vi "Save Notebook Rich Text Box.vi"(6 "Backup?":bool, 8 "Error In":errorcluster, 9 "Dialog (F)":bool, 10 "File Path Control":path, 11 ".NET Refnum in":refnum<k24>) -> (0 "Error Out":errorcluster, 1 "cancelled":bool, 2 "File Path out":path)   [LabVIEW 2019, in "Notebook.lvlib"]
uses:
  Notebook.lvlib
  System.Windows.Forms
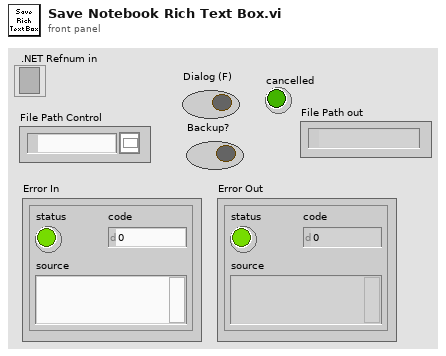
[diagram p1: front panel]
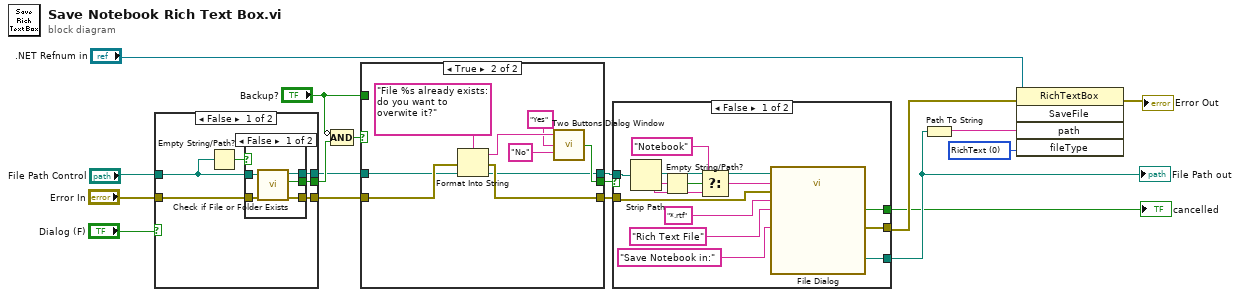
[diagram p0: block diagram]
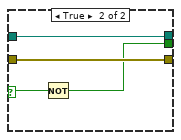
[diagram p5: hidden frame]
diagram:
  w10 = 0 items=["RichText", "PlainText", "RichNoOleObjs", "TextTextOleObjs", "UnicodePlainText"] ("fileType")
  n1 = case shown="False" "Dialog (F)" {
    selector: "Dialog (F)" -> [_ w35]
    tunnel: "File Path Control" -> [w21 w32]
    tunnel: "Error In" -> [w24 w34]
    tunnel: [w23 w34] -> w5
    tunnel: [w22 w33] -> w8
    tunnel: [w19 w32] -> w7
    frame False {
      n2 = Empty String/Path?(string/path=w21) -> (empty?=w20:bool)
      n3 = case shown="False" w20 {
        tunnel: w24 -> [w29 w31]
        tunnel: [w28 w31] -> w23
        tunnel: [w27 _] -> w22
        tunnel: w21 -> [w26 w30]
        tunnel: [w25 w30] -> w19
        frame False {
          n4 = call <vilib>:"Check if File or Folder Exists.vi"("error in (no error)"=w29, "path"=w26) -> ("error out"=w28:errorcluster, "file or folder exists?"=w27:bool, "dup path"=w25:path)  [unwired: 7 in]
        }
        frame True {
        }
      }
    }
    frame True {
      n5 = Not(x=w35) -> (.not. x?=w33:bool)
    }
  }
  n6 = Compound Arithmetic op=AND(invert "Backup?", w8) -> (w2:bool)
  n7 = case shown="True" w2 {
    tunnel: w7 -> [w38 w39]
    tunnel: [w38 w39] -> w6
    tunnel: w5 -> [w37 w44]
    tunnel: [w37 w43] -> w4
    tunnel: [w36 w40] -> w3
    tunnel: "Backup?" -> [w36 _]
    frame False {
    }
    frame True {
      n8 = Format Into String(format string="File %s already exists: do you want to overwite it?", error in=w44, w39) -> (resulting string=w45:string, error out=w43:errorcluster)  [unwired: 1 in]
      n9 = call "Two Buttons Dialog Window.vi"("Cancel Button Text"="No" ("F button name (\"Cancel\")"), "OK Button Text"="Yes" ("T button name (\"OK\")"), "Message"=w45) -> ("OK?"=w40:bool)
    }
  }
  n10 = case shown="False" w3 {
    tunnel: [w58 w60] -> w12
    tunnel: [w57 w61] -> w17
    tunnel: w6 -> [w56 w60]
    tunnel: w4 -> [w55 w61]
    tunnel: [w53 _] -> w11
    frame False {
      n11 = Strip Path(path=w56) -> (stripped path=w54:path, name=w47:string)
      n12 = Empty String/Path?(string/path=w47) -> (empty?=w50:bool)
      n13 = Select(t="Notebook" ("pattern label"), s=w50, f=w47) -> (s? t:f=w49:string)
      n14 = call "File Dialog"("start path"=w54, "prompt"="Save Notebook in:", "default name"=w49, "error in"=w55, "pattern (all files)"="*.rtf" ("pattern label"), "pattern label"="Rich Text File") -> ("selected path"=w58:path, "cancelled"=w53:bool, "error out"=w57:errorcluster)  [unwired: 6 in, 1 out]
    }
    frame True {
    }
  }
  "File Path out" <- w12
  "cancelled" <- w11
  n15 = Path To String(path=w12) -> (string=w9:string)
  n16 = invoke class="RichTextBox" method="SaveFile"(reference=".NET Refnum in", error in=w17, "path"=w9, "fileType"=w10) -> (error out=→"Error Out":errorcluster)  [unwired: 1 in, 4 out]
